vi "Digital Pattern Gen 1.3 Tooth to Edges.vi"(8 "position LUT":u16[](array[numeric]), 10 "tooth to remove":i16, 11 "first falling":bool) -> (1 "fault wrap":bool, 2 "edge 2":u16, 3 "edge 1":u16)   [LabVIEW 2013, in "Engine Simulation Toolkit Engine.lvlib"]
uses:
  Engine Simulation Toolkit Engine.lvlib
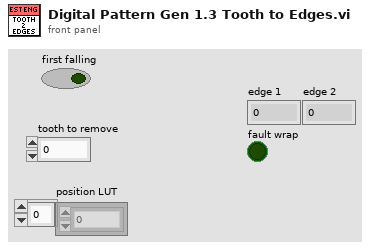
[diagram p1: front panel]
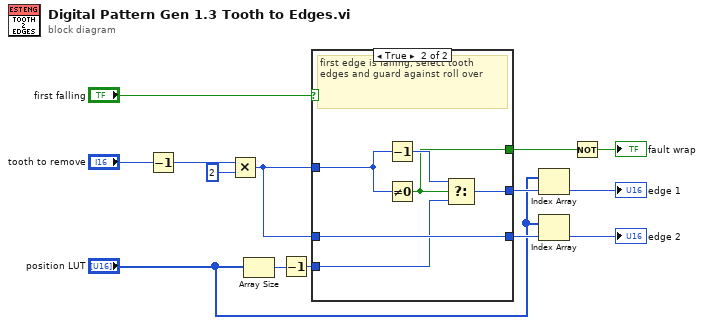
[diagram p0: block diagram]
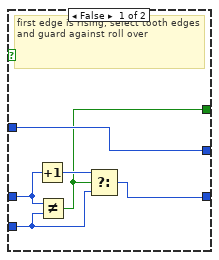
[diagram p2: hidden frame]
diagram:
  n1 = Decrement(x="tooth to remove") -> (x-1=w5:i16)
  n2 = Multiply(x=w5, y=2) -> (x*y=w13:i32)
  n3 = Array Size(array="position LUT") -> (size(s)=w11:i32)
  n4 = Decrement(x=w11) -> (x-1=w10:i32)
  n5 = case shown="True" "first falling" {
    tunnel: w13 -> [w20 w25]
    tunnel: w13 -> [w19 w26]
    tunnel: [w20 w23] -> w9
    tunnel: [w16 w26] -> w8
    tunnel: [w15 w22] -> w12
    tunnel: w10 -> [w18 w21]
    frame False {
      # "first edge is rising, select tooth edges and guard against roll over"
      n6 = Increment(x=w19) -> (x+1=w17:i32)
      n7 = Not Equal?(x=w19, y=w18) -> (x != y?=w15:bool)
      n8 = Select(t=w17, s=w15, f=w18) -> (s? t:f=w16:i32)
    }
    frame True {
      # "first edge is falling, select tooth edges and guard against roll over"
      n9 = Decrement(x=w25) -> (x-1=w24:i32)
      n10 = Not Equal To 0?(x=w25) -> (x != 0?=w22:bool)
      n11 = Select(t=w24, s=w22, f=w21) -> (s? t:f=w23:i32)
    }
  }
  n12 = Index Array(array="position LUT", index=w9) -> (element=→"edge 1":u16)
  n13 = Index Array(array="position LUT", index=w8) -> (element=→"edge 2":u16)
  n14 = Not(x=w12) -> (.not. x?=→"fault wrap":bool)
